vi "IAmGLF-SendToStandaloneProcess.vi"(8 "error in (no error)":errorcluster, 10 "Class Return Notifier":refnum<notifier>, 11 "IAmGLF in":refnum<class "IAmGLF.lvclass">) -> (0 "error out":errorcluster, 3 "IAmGLF out":refnum<class "IAmGLF.lvclass">)   [LabVIEW 2024, in "GLF.lvlib" / "IAmGLF.lvclass"]
doc: "<B>Summary</B>\nUsed to send <B>IAmGLF</B> along with <B>Data</B> to a standalone entity in order for it to create the class internal DVR.\n\n<B>Details</B>\nThis is done that way because LabVIEW automatically releases references created by VIs (or their callers) that are no longer running. So we must rely on an another asych process to be sure the DVR is not deleted."
uses:
  IAmGLF.lvclass
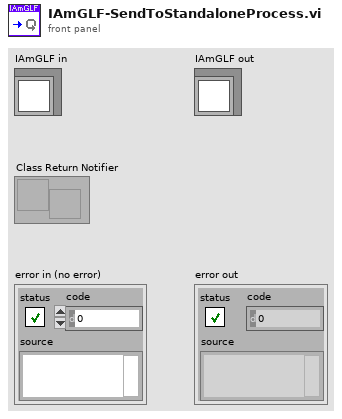
[diagram p1: front panel]
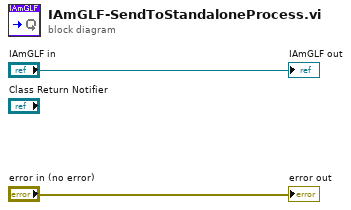
[diagram p0: block diagram]
diagram:
  "error out" <- "error in (no error)"
  "IAmGLF out" <- "IAmGLF in"
